vi "FLEnergyCheck.vi"(8 "Error In":errorcluster, 10 "delay before read (ms)":u32=500, 11 "VISA resource name":refnum<visa-resource-name>) -> (0 "Error Out":errorcluster, 1 "Write byte count":u32, 2 "Read byte count":u32, 3 "read buffer":string)   [LabVIEW 2016]
uses:
  <vilib>/Instr/_visa.llb/VISA Configure Serial Port (Instr).vi
panel:
  out "Bytes read":u32
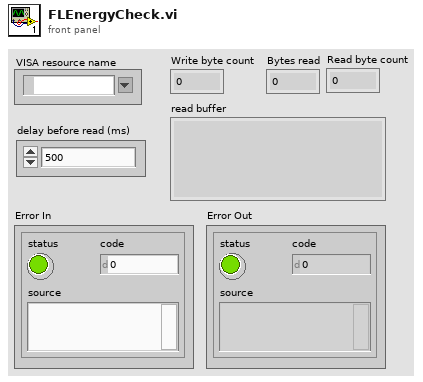
[diagram p1: front panel]
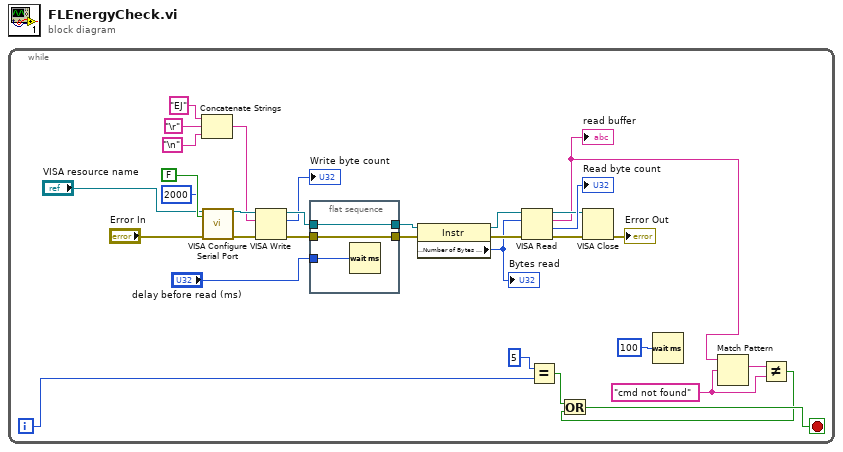
[diagram p0: block diagram]
diagram:
  n1 = while {
    i -> [w1]
    stop <- w3 stop-if-true
    w7 = "cmd not found" ("regular expression")
    n2 = Concatenate Strings("EJ" ("Command"), "\r", "\n") -> (w24:string)
    n3 = call-poly "VISA Configure Serial Port"("VISA resource name"="VISA resource name", "timeout (10sec)"=u32 2000, "Enable Termination\nChar (T)"=FALSE ("Enable Termination\nChar (T)"), "error in (no error)"="Error In") -> ("VISA resource name out"=w25:refnum<visa-resource-name>, "error out"=w23:errorcluster)  [unwired: 5 in, 5 out]
    n4 = VISA Write(VISA resource name=w25, write buffer=w24, error in (no error)=w23) -> (VISA resource name out=w21:refnum<visa-resource-name>, return count=→"Write byte count":u32, error out=w20:errorcluster)
    n5 = flat-sequence {
      tunnel: w20 -> [w34]
      tunnel: [w34] -> w18
      tunnel: w21 -> [w33]
      tunnel: [w33] -> w17
      tunnel: "delay before read (ms)" -> [w35]
      frame #0 {
        n6 = Wait (ms)(milliseconds to wait=w35) -> ()  [unwired: 1 out]
      }
    }
    n7 = property class="Instr"(reference=w17, error in=w18) -> (reference out=w13:refnum<visa-resource-name>, error out=w12:errorcluster, "Serial Settings:Number of Bytes at Serial Port"=w11:u32)
    "Bytes read" <- w11
    n8 = VISA Read(VISA resource name=w13, byte count=w11, error in (no error)=w12) -> (VISA resource name out=w15:refnum<visa-resource-name>, read buffer=w6:string, return count=→"Read byte count":u32, error out=w14:errorcluster)
    "read buffer" <- w6
    n9 = Equal?(x=5, y=w1) -> (x = y?=w4:bool)
    n10 = VISA Close(VISA resource name=w15, error in (no error)=w14) -> (error out=→"Error Out":errorcluster)
    n11 = Wait (ms)(milliseconds to wait=u32 100) -> ()  [unwired: 1 out]
    n12 = Match Pattern(string=w6, regular expression=w7) -> (match substring=w8:string)  [unwired: 1 in, 3 out]
    n13 = Not Equal?(x=w8, y=w7) -> (x != y?=w2:bool)
    n14 = Or(x=w4, y=w2) -> (x .or. y?=w3:bool)
  }
